vi "maze.vi"   [LabVIEW 2012]
uses:
  <vilib>/NXT/Subs/MotorOutput.ctl
  <vilib>/NXT/Dual Mode Library/prims/sign/sign_float.vi
  <vilib>/NXT/Dual Mode Library/Waits/Wait_Num.vi
  <vilib>/NXT/Dual Mode Library/Motors/MotorBrake.vi
types:
  T1 = typedef "MotorOutput.ctl" = u8
  T2 = typedef "LVHSConnector.ctl" = cluster{"Hardware":string, "Flattened String":string}
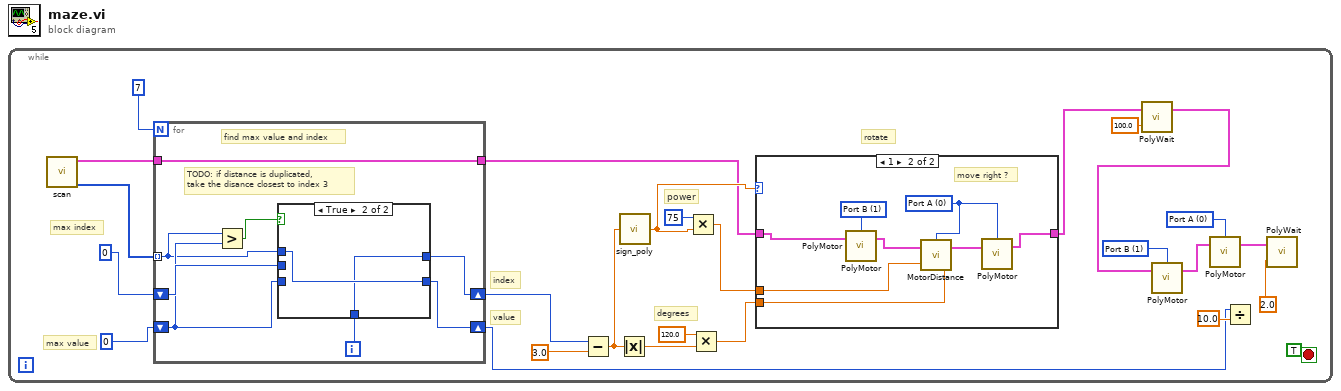
[diagram p0: block diagram]
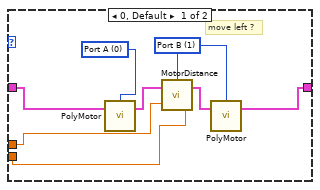
[diagram p2: hidden frame]
diagram:
  n1 = while {
    stop <- TRUE stop-if-true
    w10 = T1 0 items=["Port A"=0, "Port B"=1, "Port C"=2, "Ports A & B"=4, "Ports A & C"=5, "Ports B & C"=6, "as"=3] ("Output Port (All Ports)")
    w11 = T1 1 items=["Port A"=0, "Port B"=1, "Port C"=2, "Ports A & B"=4, "Ports A & C"=5, "Ports B & C"=6, "as"=3] ("Output Port (All Ports)")
    # "rotate"
    # "power"
    # "degrees"
    # "value"
    # "index"
    # "max value"
    # "max index"
    n2 = call "scan.vi"() -> ("Array"=w24:i32[], "NXT 2"=w25:T2)  [unwired: 10 in]
    n3 = for {
      N: 7 -> [_]
      tunnel: w25 -> [w43]
      tunnel: w24 -> [w47] mode=indexing
      shift-right: [w44] -> w17
      shift-left: 0 -> [w49]
      shift-right: [w46] -> w6
      shift-left: 0 -> [w48]
      tunnel: [w43] -> w4
      i -> [w45]
      # "TODO: if distance is duplicated,\ntake the disance closest to index 3"
      # "find max value and index"
      n4 = Greater?(x=w47, y=w48) -> (0:w50:bool)
      n5 = case shown="True" w50 {
        tunnel: w49 -> [w51 _]
        tunnel: w48 -> [w52 _]
        tunnel: w47 -> [_ w54]
        tunnel: [w52 w54] -> w46
        tunnel: w45 -> [_ w53]
        tunnel: [w51 w53] -> w44
        frame False {
        }
        frame True {
        }
      }
    }
    n6 = Subtract(x=w17, y=3.0 ("x")) -> (x-y=w16:dbl)
    n7 = Absolute Value(x=w16) -> (abs(x)=w19:dbl)
    n8 = call-poly <vilib>:"sign_poly.vi"("number"=w16) -> ("-1, 0, 1"=w14:dbl)  [unwired: 4 in]
    n9 = Multiply(x=75, y=w14) -> (x*y=w12:dbl)
    n10 = Multiply(x=120.0, y=w19) -> (x*y=w13:dbl)
    n11 = case shown="1" w14 {
      tunnel: w4 -> [w31 w38]
      tunnel: [w29 w37] -> w3
      tunnel: w13 -> [w28 w35]
      tunnel: w12 -> [w27 w36]
      frame 0, Default {
        w33 = T1 1 items=["Port A"=0, "Port B"=1, "Port C"=2, "Ports A & B"=4, "Ports A & C"=5, "Ports B & C"=6, "as"=3] ("Output Port (All Ports)")
        w34 = T1 0 items=["Port A"=0, "Port B"=1, "Port C"=2, "Ports A & B"=4, "Ports A & C"=5, "Ports B & C"=6, "as"=3] ("Output Port (All Ports)")
        # "move left ?"
        n12 = call-poly <vilib>:"PolyMotor.vi"("NXT"=w31, "Port (All Ports)"=w34) -> ("NXT"=w30:T2)  [unwired: 2 in]
        n13 = call <vilib>:"MotorDistance.vi"("Power (75)"=w27, "Angle of Rotation (360)"=w28, "NXT"=w30, "Output Port (All Ports)"=w33) -> ("NXT"=w32:T2)
        n14 = call-poly <vilib>:"PolyMotor.vi"("NXT"=w32, "Port (All Ports)"=w33) -> ("NXT"=w29:T2)  [unwired: 2 in]
      }
      frame 1 {
        w40 = T1 0 items=["Port A"=0, "Port B"=1, "Port C"=2, "Ports A & B"=4, "Ports A & C"=5, "Ports B & C"=6, "as"=3] ("Output Port (All Ports)")
        w39 = T1 1 items=["Port A"=0, "Port B"=1, "Port C"=2, "Ports A & B"=4, "Ports A & C"=5, "Ports B & C"=6, "as"=3] ("Output Port (All Ports)")
        # "move right ?"
        n15 = call-poly <vilib>:"PolyMotor.vi"() -> ()  [unwired: 4 in, 1 out]
        n16 = call-poly <vilib>:"PolyMotor.vi"("NXT"=w38, "Port (All Ports)"=w39) -> ("NXT"=w42:T2)  [unwired: 2 in]
        n17 = call <vilib>:"MotorDistance.vi"("Power (75)"=w36, "Angle of Rotation (360)"=w35, "NXT"=w42, "Output Port (All Ports)"=w40) -> ("NXT"=w41:T2)
        n18 = call-poly <vilib>:"PolyMotor.vi"("NXT"=w41, "Port (All Ports)"=w40) -> ("NXT"=w37:T2)  [unwired: 2 in]
      }
    }
    n19 = call-poly <vilib>:"PolyWait.vi"("Time (1 sec)"=100.0 ("x"), "NXT"=w3) -> ("NXT"=w2:T2)  [unwired: 2 in]
    n20 = call-poly <vilib>:"PolyMotor.vi"("NXT"=w2, "Port (All Ports)"=w11) -> ("NXT"=w9:T2)  [unwired: 2 in]
    n21 = call-poly <vilib>:"PolyMotor.vi"("NXT"=w9, "Port (All Ports)"=w10) -> ("NXT"=w8:T2)  [unwired: 2 in]
    n22 = Divide(x=w6, y=10.0 ("x")) -> ()  [unwired: 1 out]
    n23 = call-poly <vilib>:"PolyWait.vi"("Time (1 sec)"=2.0 ("x"), "NXT"=w8) -> ()  [unwired: 2 in, 1 out]
  }
